vi "dvr exists.vi"(8 "error in (no error)":errorcluster) -> (0 "error out":errorcluster, 3 "exists":bool)   [LabVIEW 2024, in "controls manager.lvlib"]
uses:
  controls manager.lvlib
  fgv actions.ctl
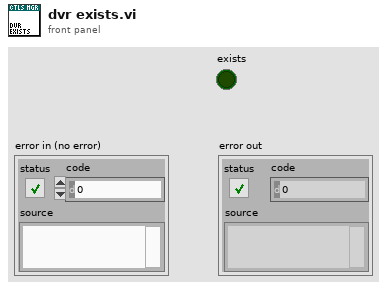
[diagram p1: front panel]
types:
  T1 = typedef "controls manager.lvlib/fgv actions.ctl" = enum16{"create", "get", "destroy"}
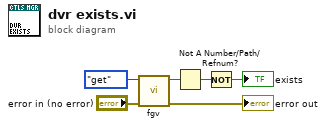
[diagram p0: block diagram]
diagram:
  n1 = call "fgv.vi"("error in (no error)"="error in (no error)", "action"=fgv_actions."get") -> ("error out"=→"error out":errorcluster, "dvr"=w6:refnum<data-value>)  [unwired: 8 in]
  n2 = Not A Number/Path/Refnum?(number/path/refnum=w6) -> (NaN/Path/Refnum?=w3:bool)
  n3 = Not(x=w3) -> (.not. x?=→"exists":bool)
